vi "zad3.vi"() -> ()   [LabVIEW 2017]
panel:
  out "Alarm":bool
  out "Numeric":i32
  out "millisecond timer value 2":u32[](array[numeric])
  out "millisecond timer value":u32[](array[numeric])
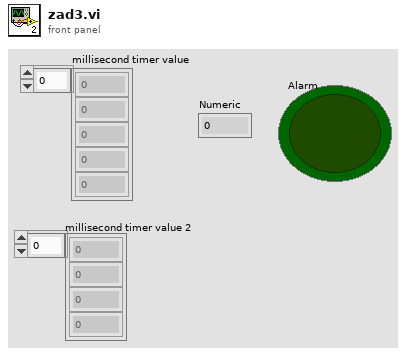
[diagram p1: front panel]
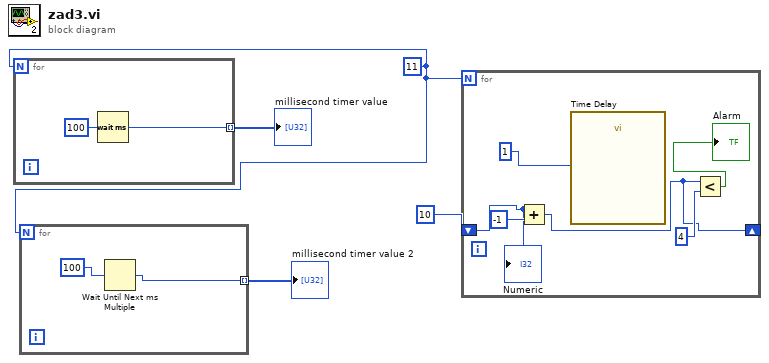
[diagram p0: block diagram]
diagram:
  w2 = 11
  n1 = for {
    N: w2 -> [_]
    tunnel: [w5] -> w4 mode=indexing
    n2 = Wait (ms)(milliseconds to wait=u32 100) -> (millisecond timer value=w5:u32)
  }
  "millisecond timer value" <- w4
  n3 = for {
    N: w2 -> [_]
    tunnel: [w7] -> w3 mode=indexing
    n4 = Wait Until Next ms Multiple(millisecond multiple=u32 100 ("milliseconds to wait")) -> (millisecond timer value=w7:u32)
  }
  "millisecond timer value 2" <- w3
  n5 = for {
    N: w2 -> [_]
    shift-right: [w10] -> _
    shift-left: 10 -> [w12]
    n6 = Add(x=w12, y=-1) -> (x+y=w10:i32)
    n7 = call "Time Delay"("Delay Time (s)"=u32 1 ("milliseconds to wait")) -> ()  [unwired: 10 in, 1 out]
    n8 = Less?(x=w10, y=4) -> (x < y?=→"Alarm":bool)
    "Numeric" <- w12
  }
